vi "Update Configuration MCL.vi"(5 "number of RTD input channels":i32=8, 6 "error in":errorcluster, 7 "_9226 Config":T2 {"RTD_Type" items=["User Defined"=0, "TCR3750"=2, "TCR3851"=7]; "Degree Range" items=["Raw Ohms", "Degrees Kelvin", "Degrees Celsius", "Degrees Fahrenheit", "Degrees Rankine"]; "Conversion Time" items=["200 ms", "2.5 ms"]}, 9 "_Channel Refnum":refnum<vi>) -> (0 "error out":errorcluster)   [LabVIEW 2019, in "Modules.lvlib" / "9226.lvclass"]
uses:
  9226.lvclass
  9226 Configuration.ctl
  Supported RTD Types.ctl
panel:
  in  "RTD type":T1=2 items=["Custom"=0, "TCR3750"=2, "TCR3851"=7]
  in  "Degree Range":u32(ring) items=["Raw Ohms", "Degrees Kelvin", "Degrees Celsius", "Degrees Fahrenheit", "Degrees Rankine"]
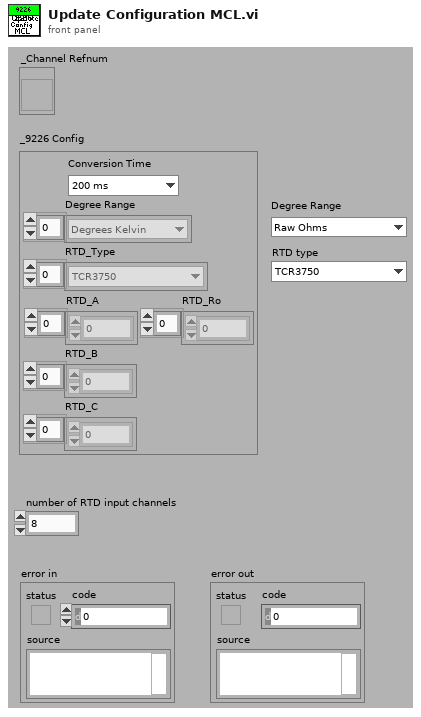
[diagram p1: front panel]
types:
  T1 = typedef "Modules.lvlib/9226.lvclass/Supported RTD Types.ctl" = u32
  T2 = typedef "Modules.lvlib/9226.lvclass/9226 Configuration.ctl" = cluster{"Conversion Time":u16, "Degree Range":u32[], "RTD_Type":T1[], "RTD_A":dbl[], "RTD_B":dbl[], "RTD_C":dbl[], "RTD_Ro":dbl[]}
  T3 = typedef "LVStringsAndValuesArrayTypeDef_U32.ctl" = cluster{"String":string, "Value":u32}[]
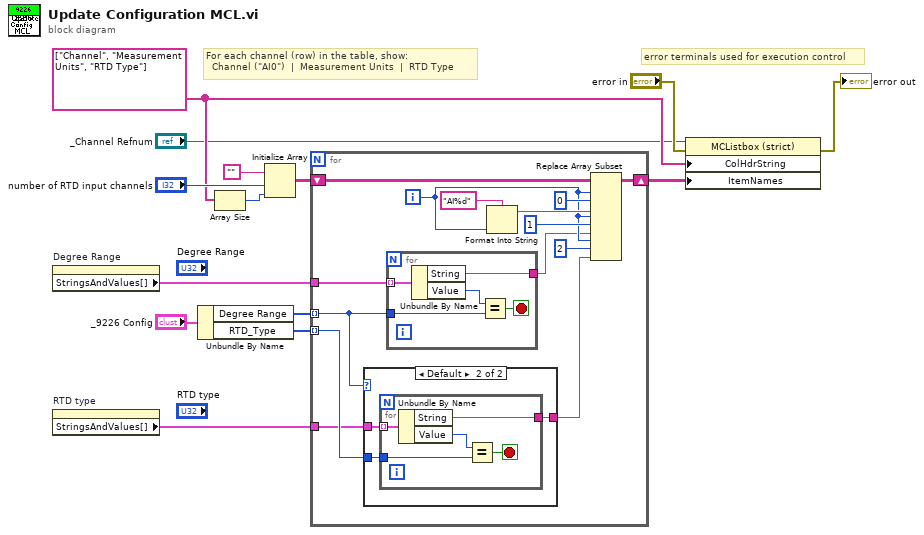
[diagram p0: block diagram]
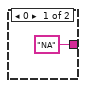
[diagram p2: hidden frame]
diagram:
  w5 = string[] ["Channel", "Measurement Units", "RTD Type"]
  # "For each channel (row) in the table, show:\n  Channel (\"AI0\")  |  Measurement Units  |  RTD Type"
  # "error terminals used for execution control"
  n1 = property on="Degree Range" class="Ring (strict)"() -> ("StringsAndValues[]"=w8:T3)  [unwired: 2 in, 2 out]
  n2 = property on="RTD type" class="Ring (strict)"() -> ("StringsAndValues[]"=w9:T3)  [unwired: 2 in, 2 out]
  n3 = Unbundle By Name("_9226 Config") -> ("Degree Range"=w7:u32[], "RTD_Type"=w10:T1[])
  n4 = Array Size(array=w5) -> (size(s)=w4:i32)
  n5 = Initialize Array("", "number of RTD input channels", w4) -> (w14:string[][])
  n6 = for {
    shift-right: [w27] -> w6
    shift-left: w14 -> [w26]
    tunnel: w10 -> [w19] mode=indexing
    tunnel: w7 -> [w15] mode=indexing
    tunnel: w9 -> [w17]
    tunnel: w8 -> [w16]
    i -> [w22]
    n7 = case shown="Default" w15 {
      tunnel: w19 -> [_ w32]
      tunnel: ["NA" ("Section") w31] -> w18
      tunnel: w17 -> [_ w30]
      frame 0 {
      }
      frame Default {
        n8 = for {
          tunnel: w30 -> [w37] mode=indexing
          tunnel: w32 -> [w35]
          tunnel: [w33] -> w31
          stop <- w34 stop-if-true
          n9 = Unbundle By Name(w37) -> ("String"=w33:string, "Value"=w36:u32)
          n10 = Equal?(x=w36, y=w35) -> (x = y?=w34:bool)
        }
      }
    }
    n11 = for {
      tunnel: w16 -> [w42] mode=indexing
      tunnel: w15 -> [w40]
      tunnel: [w38] -> w20
      stop <- w39 stop-if-true
      n12 = Unbundle By Name(w42) -> ("String"=w38:string, "Value"=w41:u32)
      n13 = Equal?(x=w41, y=w40) -> (x = y?=w39:bool)
    }
    n14 = Format Into String(format string="AI%d", w22) -> (resulting string=w23:string)  [unwired: 2 in, 1 out]
    n15 = Replace Array Subset(array=w26, new element #1=w23, index (row) #1=w22, index (col) #1=0 ("Column 1"), new element #2=w20, index (row) #2=w22, index (col) #2=1 ("Column 1"), new element #3=w18, index (row) #3=w22, index (col) #3=2 ("disabled index (col)")) -> (w27:string[][])
  }
  n16 = property on="Property Node" class="MCListbox (strict)"(reference="_Channel Refnum", error in="error in", "ColHdrString"=w5, "ItemNames"=w6) -> (error out=→"error out":errorcluster)  [unwired: 1 out]
